vi "intefrace.vi"() -> ()   [LabVIEW 2018]
uses:
  <vilib>/Instr/_visa.llb/VISA Configure Serial Port (Instr).vi
panel:
  in  "VISA resource name":refnum<visa-resource-name>
  out "Regador":bool
  out "Termómetro (°C)":dbl(slide) scale=0.0..100.0
  out "Humedad del aire (%)":dbl(knob) scale=0.0..100.0
  out "Humedad del agua (%)":dbl(knob) scale=0.0..100.0
  out "Lectura de datos":string
  out "Mensajes de error":errorcluster
  in  "Botón de ALTO":bool
  in  "Ruta del archivo de datos":path
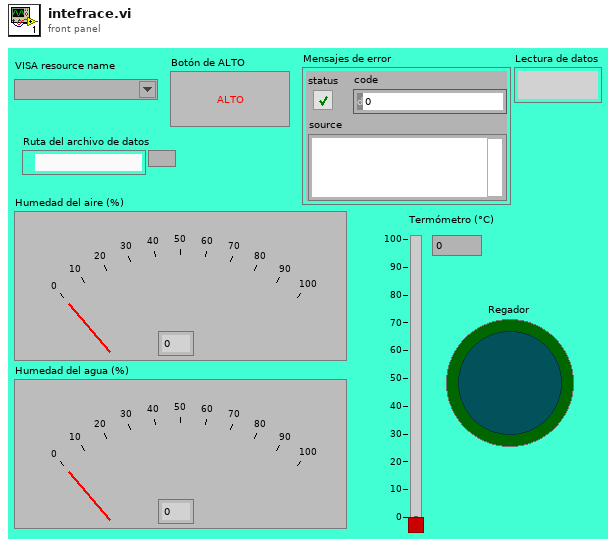
[diagram p1: front panel]
types:
  T1 = enum16{"open", "replace", "create", "open or create", "replace or create", "replace or create with confirmation"}
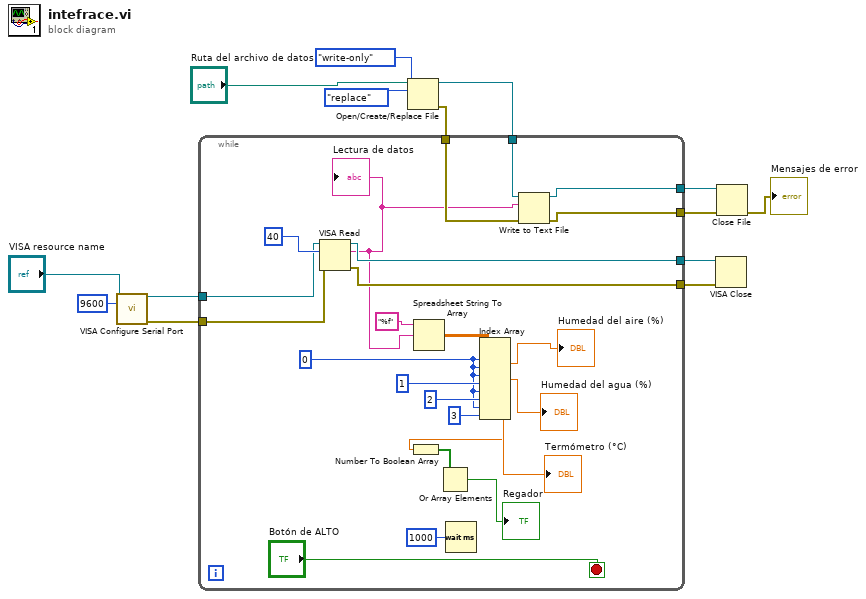
[diagram p0: block diagram]
diagram:
  n1 = call-poly "VISA Configure Serial Port"("VISA resource name"="VISA resource name", "baud rate (9600)"=u32 9600) -> ("VISA resource name out"=w4:refnum<visa-resource-name>, "error out"=w3:errorcluster)  [unwired: 12 in]
  n2 = Open/Create/Replace File(file path (use dialog)="Ruta del archivo de datos", operation (0:open)=T1."replace", access (0:read/write)=enum16{"read/write", "read-only", "write-only"}."write-only") -> (refnum out=w10:refnum<file>, error out=w11:errorcluster)  [unwired: 3 in, 1 out]
  n3 = while {
    tunnel: w11 -> [w35]
    tunnel: w10 -> [w34]
    tunnel: [w33] -> w9
    tunnel: [w32] -> w8
    tunnel: [w31] -> w6
    tunnel: [w30] -> w5
    tunnel: w4 -> [w16]
    tunnel: w3 -> [w15]
    stop <- "Botón de ALTO" stop-if-true
    w21 = 0 ("index (row)")
    n4 = VISA Read(VISA resource name=w16, byte count=u32 40, error in (no error)=w15) -> (VISA resource name out=w31:refnum<visa-resource-name>, read buffer=w28:string, error out=w30:errorcluster)  [unwired: 1 out]
    "Lectura de datos" <- w28
    n5 = Spreadsheet String To Array(format string="%f", spreadsheet string=w28) -> (array=w27:dbl[][])  [unwired: 2 in]
    n6 = Wait (ms)(milliseconds to wait=u32 1000) -> ()  [unwired: 1 out]
    n7 = Index Array(array=w27, index (row) #1=w21, index (col) #1=w21, index (row) #2=w21, index (col) #2=1 ("disabled index (col)"), index (row) #3=w21, index (col) #3=2 ("disabled index (col)"), index (row) #4=w21, index (col) #4=3 ("disabled index (col)")) -> (element #1=→"Humedad del aire (%)":dbl, element #2=→"Humedad del agua (%)":dbl, element #3=→"Termómetro (°C)":dbl, element #4=w19:dbl)
    n8 = Number To Boolean Array(number=w19) -> (Boolean array=w18:bool[])
    n9 = Or Array Elements(Boolean array=w18) -> (logical OR=→"Regador":bool)
    n10 = Write to Text File(file (use dialog)=w34, text=w28, error in=w35) -> (refnum out=w33:refnum<file>, error out=w32:errorcluster)  [unwired: 1 in, 1 out]
  }
  n11 = VISA Close(VISA resource name=w6, error in (no error)=w5) -> ()  [unwired: 1 out]
  n12 = Close File(refnum=w9, error in=w8) -> (error out=→"Mensajes de error":errorcluster)  [unwired: 1 out]
